vi "Notify and Filter Events.vi"() -> ()   [LabVIEW 2015]
panel:
  in  "Stop":bool
  out "Current Date and Time":timestamp format="%<%x %X>T"
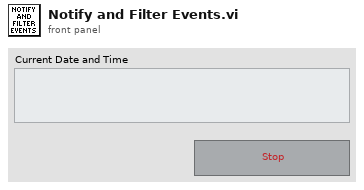
[diagram p1: front panel]
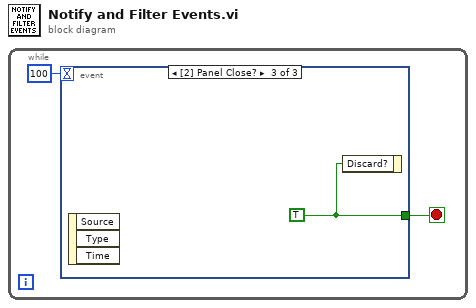
[diagram p0: block diagram]
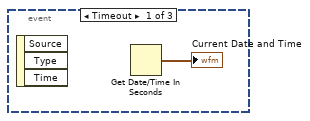
[diagram p2: hidden frame]
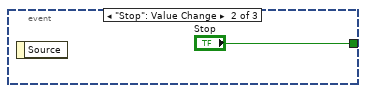
[diagram p3: hidden frame]
diagram:
  n1 = while {
    stop <- w1 stop-if-true
    n2 = event shown="[2] Panel Close?" {
      selector: _ -> [_ _ _]
      dyn-events: _ -> [_ _ _]
      timeout: 100 -> [_ _ _]
      tunnel: [_ "Stop" w5] -> w1
      event Timeout {
        n3 = event-data() -> ()  [unwired: 1 in, 3 out]
        n4 = Get Date/Time In Seconds() -> (seconds since 1Jan1904=→"Current Date and Time":timestamp)
      }
      event "Stop": Value Change {
        n5 = event-data() -> ()  [unwired: 1 in, 1 out]
      }
      event Panel Close? {
        w5 = TRUE ("Stop")
        n6 = event-data() -> ()  [unwired: 1 in, 3 out]
        n7 = event-data("Discard?"=w5) -> ()  [unwired: 1 in, 1 out]
      }
    }
  }
